vi "Dynamic Event Handler.vi"() -> ()   [LabVIEW 2013, in "Interaction By Refererence.lvclass"]
uses:
  Interaction By Refererence.lvclass
  Interaction By Refererence.lvclass/Interaction By Refererence.ctl
  IContainer/Interaction/Interaction.lvclass
panel:
  in  "Numeric 2":i32
  in  "Numeric":i32
  in  "Interaction":refnum<class "Interaction By Refererence.lvclass">
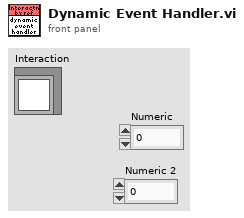
[diagram p1: front panel]
types:
  T1 = enum32{"Bad", "Idle", "Run top level", "Running"}
  T2 = typedef "LVRectTypeDef.ctl" = cluster{"Left":i16, "Top":i16, "Right":i16, "Bottom":i16}
  T3 = enum16{"VK_LBUTTON", "VK_RBUTTON", "VK_CANCEL", "VK_MBUTTON", "VK_XBUTTON1", "VK_XBUTTON2", "0x07", "VK_BACK", "VK_TAB", "0x0A", "0x0B", "VK_CLEAR", "VK_RETURN", "0x0E", "0x0F", "VK_SHIFT", "VK_CONTROL", "VK_MENU", "VK_PAUSE", "VK_CAPITAL", "VK_KANA\\VK_HANGUL", "0x16", "VK_JUNJA", "VK_FINAL", "VK_HANJA\\VK_KANJI", "0x1A", "VK_ESCAPE", "VK_CONVERT", "VK_NONCONVERT", "VK_ACCEPT", "VK_MODECHANGE", "VK_SPACE", "VK_PRIOR", "VK_NEXT", "VK_END", "VK_HOME", "VK_LEFT", "VK_UP", "VK_RIGHT", "VK_DOWN", "VK_SELECT", "VK_PRINT", "VK_EXECUTE", "VK_SNAPSHOT", "VK_INSERT", "VK_DELETE", "VK_HELP", "0 key", "1 key", "2 key", "3 key", "4 key", "5 key", "6 key", "7 key", "8 key", "9 key", "0x3A", "0x3B", "0x3C", "0x3D", "0x3E", "0x3F", "0x40", "A key", "B key", "C key", "D key", "E key", "F key", "G key", "H key", "I key", "J key", "K key", "L key", "M key", "N key", "O key", "P key", "Q key", "R key", "S key", "T key", "U key", "V key", "W key", "X key", "Y key", "Z key", "VK_LWIN", "VK_RWIN", "VK_APPS", "0x5E", "VK_SLEEP", "VK_NUMPAD0", "VK_NUMPAD1", "VK_NUMPAD2", "VK_NUMPAD3", "VK_NUMPAD4", "VK_NUMPAD5", "VK_NUMPAD6", "VK_NUMPAD7", "VK_NUMPAD8", "VK_NUMPAD9", "VK_MULTIPLY", "VK_ADD", "VK_SEPARATOR", "VK_SUBTRACT", "VK_DECIMAL", "VK_DIVIDE", "VK_F1", "VK_F2", "VK_F3", "VK_F4", "VK_F5", "VK_F6", "VK_F7", "VK_F8", "VK_F9", "VK_F10", "VK_F11", "VK_F12", "VK_F13", "VK_F14", "VK_F15", "VK_F16", "VK_F17", "VK_F18", "VK_F19", "VK_F20", "VK_F21", "VK_F22", "VK_F23", "VK_F24", "0x88", "0x89", "0x8A", "0x8B", "0x8C", "0x8D", "0x8E", "0x8F", "VK_NUMLOCK", "VK_SCROLL", "0x92", "0x93", "0x94", "0x95", "0x96", "0x97", "0x98", "0x99", "0x9A", "0x9B", "0x9C", "0x9D", "0x9E", "0x9F", "VK_LSHIFT", "VK_RSHIFT", "VK_LCONTROL", "VK_RCONTROL", "VK_LMENU", "VK_RMENU", "VK_BROWSER_BACK", "VK_BROWSER_FORWARD", "VK_BROWSER_REFRESH", "VK_BROWSER_STOP", "VK_BROWSER_SEARCH", "VK_BROWSER_FAVORITES", "VK_BROWSER_HOME", "VK_VOLUME_MUTE", "VK_VOLUME_DOWN", "VK_VOLUME_UP", "VK_MEDIA_NEXT_TRACK", "VK_MEDIA_PREV_TRACK", "VK_MEDIA_STOP", "VK_MEDIA_PLAY_PAUSE", "VK_LAUNCH_MAIL", "VK_LAUNCH_MEDIA_SELECT", "VK_LAUNCH_APP1", "VK_LAUNCH_APP2", "0xB8", "0xB9", "VK_OEM_1", "VK_OEM_PLUS", "VK_OEM_COMMA", "VK_OEM_MINUS", "VK_OEM_PERIOD", "VK_OEM_2", "VK_OEM_3", "0xC1", "0xC2", "0xC3", "0xC4", "0xC5", "0xC6", "0xC7", "0xC8", "0xC9", "0xCA", "0xCB", "0xCC", "0xCD", "0xCE", "0xCF", "0xD0", "0xD1", "0xD2", "0xD3", "0xD4", "0xD5", "0xD6", "0xD7", "0xD8", "0xD9", "0xDA", "VK_OEM_4", "VK_OEM_5", "VK_OEM_6", "VK_OEM_7", "VK_OEM_8", "0xE0", "0xE1", "VK_OEM_102", "0xE3", "0xE4", "VK_PROCESSKEY", "0xE6", "VK_PACKET", "0xE7", "0xE8", "0xE9", "0xEA", "0xEB", "0xEC", "0xED", "0xEF", "0xF0", "0xF1", "0xF2", "0xF3", "0xF4", "0xF5", "VK_ATTN", "VK_CRSEL", "VK_EXSEL", "VK_EREOF", "VK_PLAY", "VK_ZOOM", "VK_NONAME", "VK_PA1", "VK_OEM_CLEAR"}[]
  T4 = typedef "LVPoint32TypeDef.ctl" = cluster{"Horizontal":i32, "Vertical":i32}
  T5 = typedef "sizeaction.ctl" = enum32{"Minimized", "Maximized", "Resized"}
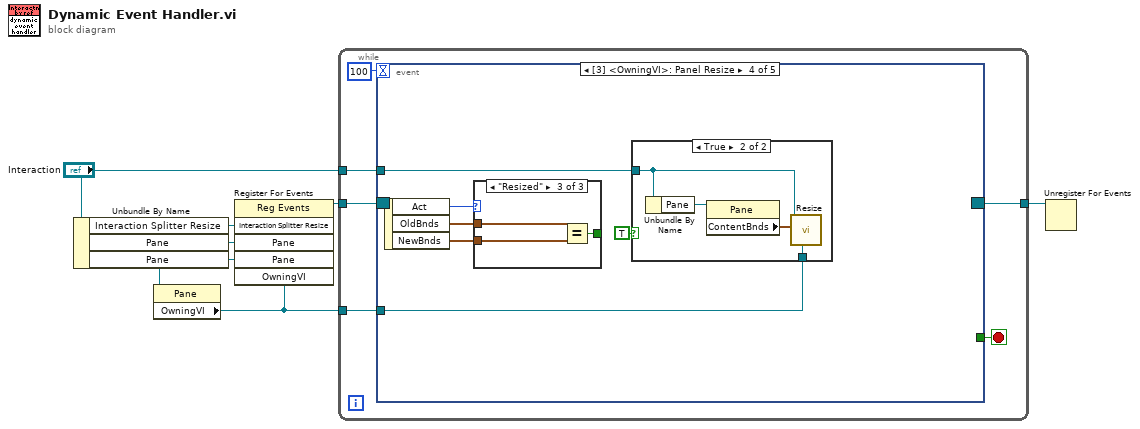
[diagram p0: block diagram]
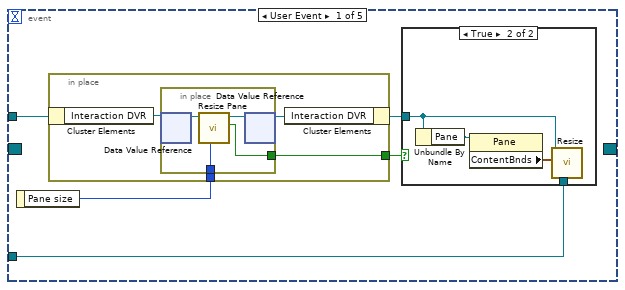
[diagram p2: hidden frame]
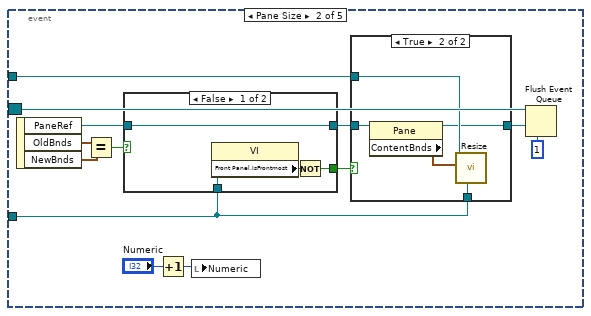
[diagram p4: hidden frame]
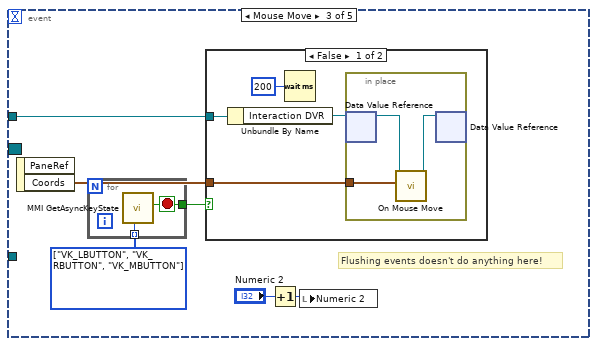
[diagram p7: hidden frame]
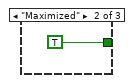
[diagram p11: hidden frame]
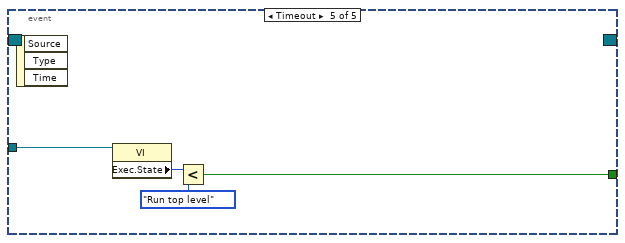
[diagram p12: hidden frame]
diagram:
  n1 = Unbundle By Name("Interaction") -> ("Interaction Splitter Resize"=w7:refnum<user-event>, "Pane"=w4:refnum<vi>, "Pane"=w3:refnum<vi>)
  n2 = property class="Pane"(reference=w3) -> ("OwningVI"=w2:refnum<vi>)  [unwired: 1 in, 2 out]
  n3 = register-events(w7, w4, w3, w2) -> (reference out=w6:refnum<event-registration>)  [unwired: 2 in, 1 out]
  n4 = while {
    tunnel: w6 -> [w12]
    tunnel: "Interaction" -> [w11]
    tunnel: w2 -> [w10]
    tunnel: [w8] -> w1
    stop <- w13 stop-if-true
    n5 = event shown="[3] <OwningVI>: Panel Resize" {
      selector: w12 -> [_ w36 _ _ _]
      dyn-events: [_ _ _ _ _] -> w8
      timeout: 100 -> [_ _ _ _ _]
      tunnel: [_ _ _ _ w85] -> w13
      tunnel: w11 -> [w16 w40 w59 w76 _]
      tunnel: w10 -> [w14 w31 _ w72 w88]
      event User Event {
        n6 = event-data() -> ("Pane size"=w15:i32)  [unwired: 1 in]
        n7 = in-place {
          in-place-border: [w22] -> w17
          in-place-border: w15 -> [w19]
          n8 = in-place-cluster #1(w16) -> ("Interaction DVR"=w20:refnum<data-value>)
          n9 = in-place {
            in-place-border: [w26] -> w22
            in-place-border: w19 -> [w23]
            n10 = in-place-dvr #2(w20) -> (w25:refnum<class "Interaction.lvclass">)  [unwired: 1 out]
            n11 = call-dynamic "Resize Pane.vi"("Pane size"=w23, "IContainer in"=w25) -> ("Resized?"=w26:bool, "IContainer out"=w24:refnum<class "Interaction.lvclass">)  [unwired: 7 in, 1 out]
            n12 = in-place-dvr #2(w24) -> (w21:refnum<data-value>)  [unwired: 1 out]
          }
          n13 = in-place-cluster #1("Interaction DVR"=w21) -> (w18:refnum<class "Interaction By Refererence.lvclass">)
        }
        n14 = case shown="True" w17 {
          tunnel: w18 -> [_ w29]
          tunnel: w14 -> [_ w27]
          frame False {
          }
          frame True {
            n15 = Unbundle By Name(w29) -> ("Pane"=w28:refnum<vi>)
            n16 = property on="Property Node" class="Pane"(reference=w28) -> ("ContentBnds"=w30:T2)  [unwired: 1 in, 2 out]
            n17 = call-dynamic "Resize.vi"("VI Refnum"=w27, "Bounds"=w30, "MMI Scaling in"=w29) -> ()  [unwired: 6 in, 3 out]
          }
        }
      }
      event Pane Size {
        n18 = event-data() -> ("PaneRef"=w37:refnum<vi>, "OldBnds"=w39:T2, "NewBnds"=w38:T2)  [unwired: 1 in]
        n19 = Equal?(x=w39, y=w38) -> (x = y?=w42:bool)
        n20 = case shown="False" w42 {
          selector: w42 -> [_ w49]
          tunnel: w37 -> [w44 w48]
          tunnel: [w44 w48] -> w41
          tunnel: [w47 w49] -> w43
          tunnel: w31 -> [w45 _]
          frame False {
            n21 = property on="Property Node" class="VI"(reference=w45) -> ("Front Panel.IsFrontmost"=w46:bool)  [unwired: 1 in, 2 out]
            n22 = Not(x=w46) -> (.not. x?=w47:bool)
          }
          frame True {
          }
        }
        n23 = Increment(x="Numeric") -> (x+1=w32:i32)
        n24 = local write "Numeric"(w32) -> ()
        n25 = case shown="True" w43 {
          tunnel: w40 -> [_ w53]
          tunnel: w41 -> [w50 w54]
          tunnel: [w50 w52] -> w34
          tunnel: w31 -> [_ w51]
          frame False {
          }
          frame True {
            n26 = property on="Property Node" class="Pane"(reference=w54) -> (reference out=w52:refnum<vi>, "ContentBnds"=w55:T2)  [unwired: 1 in, 1 out]
            n27 = call-dynamic "Resize.vi"("VI Refnum"=w51, "Bounds"=w55, "MMI Scaling in"=w53) -> ()  [unwired: 6 in, 3 out]
          }
        }
        n28 = Flush Event Queue(0:w36, 2:w34, 5:1 ("keep most recent")) -> ()  [unwired: 3 in, 3 out]
      }
      event Mouse Move {
        w61 = T3 [enum."VK_LBUTTON", enum."VK_RBUTTON", enum."VK_MBUTTON"] items=["VK_LBUTTON", "VK_RBUTTON", "VK_CANCEL", "VK_MBUTTON", "VK_XBUTTON1", "VK_XBUTTON2", "0x07", "VK_BACK", "VK_TAB", "0x0A", "0x0B", "VK_CLEAR", "VK_RETURN", "0x0E", "0x0F", "VK_SHIFT", "VK_CONTROL", "VK_MENU", "VK_PAUSE", "VK_CAPITAL", "VK_KANA\\VK_HANGUL", "0x16", "VK_JUNJA", "VK_FINAL", "VK_HANJA\\VK_KANJI", "0x1A", "VK_ESCAPE", "VK_CONVERT", "VK_NONCONVERT", "VK_ACCEPT", "VK_MODECHANGE", "VK_SPACE", "VK_PRIOR", "VK_NEXT", "VK_END", "VK_HOME", "VK_LEFT", "VK_UP", "VK_RIGHT", "VK_DOWN", "VK_SELECT", "VK_PRINT", "VK_EXECUTE", "VK_SNAPSHOT", "VK_INSERT", "VK_DELETE", "VK_HELP", "0 key", "1 key", "2 key", "3 key", "4 key", "5 key", "6 key", "7 key", "8 key", "9 key", "0x3A", "0x3B", "0x3C", "0x3D", "0x3E", "0x3F", "0x40", "A key", "B key", "C key", "D key", "E key", "F key", "G key", "H key", "I key", "J key", "K key", "L key", "M key", "N key", "O key", "P key", "Q key", "R key", "S key", "T key", "U key", "V key", "W key", "X key", "Y key", "Z key", "VK_LWIN", "VK_RWIN", "VK_APPS", "0x5E", "VK_SLEEP", "VK_NUMPAD0", "VK_NUMPAD1", "VK_NUMPAD2", "VK_NUMPAD3", "VK_NUMPAD4", "VK_NUMPAD5", "VK_NUMPAD6", "VK_NUMPAD7", "VK_NUMPAD8", "VK_NUMPAD9", "VK_MULTIPLY", "VK_ADD", "VK_SEPARATOR", "VK_SUBTRACT", "VK_DECIMAL", "VK_DIVIDE", "VK_F1", "VK_F2", "VK_F3", "VK_F4", "VK_F5", "VK_F6", "VK_F7", "VK_F8", "VK_F9", "VK_F10", "VK_F11", "VK_F12", "VK_F13", "VK_F14", "VK_F15", "VK_F16", "VK_F17", "VK_F18", "VK_F19", "VK_F20", "VK_F21", "VK_F22", "VK_F23", "VK_F24", "0x88", "0x89", "0x8A", "0x8B", "0x8C", "0x8D", "0x8E", "0x8F", "VK_NUMLOCK", "VK_SCROLL", "0x92", "0x93", "0x94", "0x95", "0x96", "0x97", "0x98", "0x99", "0x9A", "0x9B", "0x9C", "0x9D", "0x9E", "0x9F", "VK_LSHIFT", "VK_RSHIFT", "VK_LCONTROL", "VK_RCONTROL", "VK_LMENU", "VK_RMENU", "VK_BROWSER_BACK", "VK_BROWSER_FORWARD", "VK_BROWSER_REFRESH", "VK_BROWSER_STOP", "VK_BROWSER_SEARCH", "VK_BROWSER_FAVORITES", "VK_BROWSER_HOME", "VK_VOLUME_MUTE", "VK_VOLUME_DOWN", "VK_VOLUME_UP", "VK_MEDIA_NEXT_TRACK", "VK_MEDIA_PREV_TRACK", "VK_MEDIA_STOP", "VK_MEDIA_PLAY_PAUSE", "VK_LAUNCH_MAIL", "VK_LAUNCH_MEDIA_SELECT", "VK_LAUNCH_APP1", "VK_LAUNCH_APP2", "0xB8", "0xB9", "VK_OEM_1", "VK_OEM_PLUS", "VK_OEM_COMMA", "VK_OEM_MINUS", "VK_OEM_PERIOD", "VK_OEM_2", "VK_OEM_3", "0xC1", "0xC2", "0xC3", "0xC4", "0xC5", "0xC6", "0xC7", "0xC8", "0xC9", "0xCA", "0xCB", "0xCC", "0xCD", "0xCE", "0xCF", "0xD0", "0xD1", "0xD2", "0xD3", "0xD4", "0xD5", "0xD6", "0xD7", "0xD8", "0xD9", "0xDA", "VK_OEM_4", "VK_OEM_5", "VK_OEM_6", "VK_OEM_7", "VK_OEM_8", "0xE0", "0xE1", "VK_OEM_102", "0xE3", "0xE4", "VK_PROCESSKEY", "0xE6", "VK_PACKET", "0xE7", "0xE8", "0xE9", "0xEA", "0xEB", "0xEC", "0xED", "0xEF", "0xF0", "0xF1", "0xF2", "0xF3", "0xF4", "0xF5", "VK_ATTN", "VK_CRSEL", "VK_EXSEL", "VK_EREOF", "VK_PLAY", "VK_ZOOM", "VK_NONAME", "VK_PA1", "VK_OEM_CLEAR"]
        # "Flushing events doesn't do anything here!"
        n29 = event-data() -> ("Coords"=w58:T4)  [unwired: 1 in, 1 out]
        n30 = for {
          tunnel: [w63] -> w60
          tunnel: w61 -> [w62] mode=indexing
          stop <- w63 stop-if-true
          n31 = call "MMI GetAsyncKeyState.vi"("Enum"=w62) -> ("Pressed?"=w63:bool)  [unwired: 8 in, 2 out]
        }
        n32 = case shown="False" w60 {
          tunnel: w59 -> [w67 _]
          tunnel: w58 -> [w65 _]
          frame False {
            n33 = Unbundle By Name(w67) -> ("Interaction DVR"=w66:refnum<data-value>)
            n34 = Wait (ms)(milliseconds to wait=u32 200) -> ()  [unwired: 1 out]
            n35 = in-place {
              in-place-border: w65 -> [w70]
              n36 = in-place-dvr #3(w66) -> (w69:refnum<class "Interaction.lvclass">)  [unwired: 1 out]
              n37 = call "On Mouse Move.vi"("Coords"=w70, "Interaction in"=w69) -> ("Interaction out"=w68:refnum<class "Interaction.lvclass">)  [unwired: 8 in, 1 out]
              n38 = in-place-dvr #3(w68) -> ()  [unwired: 2 out]
            }
          }
          frame True {
          }
        }
        n39 = Increment(x="Numeric 2") -> (x+1=w56:i32)
        n40 = local write "Numeric 2"(w56) -> ()
      }
      event Panel Resize {
        n41 = event-data() -> ("Act"=w75:T5, "OldBnds"=w74:T2, "NewBnds"=w73:T2)  [unwired: 1 in]
        n42 = case shown="\"Resized\"" w75 {
          tunnel: [_ TRUE w84] -> _
          tunnel: w74 -> [_ _ w83]
          tunnel: w73 -> [_ _ w82]
          frame Default {
          }
          frame "Maximized" {
          }
          frame "Resized" {
            n43 = Equal?(x=w83, y=w82) -> (x = y?=w84:bool)
          }
        }
        n44 = case shown="True" TRUE {
          tunnel: w76 -> [_ w78]
          tunnel: w72 -> [_ w77]
          frame False {
          }
          frame True {
            n45 = Unbundle By Name(w78) -> ("Pane"=w79:refnum<vi>)
            n46 = property on="Property Node" class="Pane"(reference=w79) -> ("ContentBnds"=w80:T2)  [unwired: 1 in, 2 out]
            n47 = call-dynamic "Resize.vi"("VI Refnum"=w77, "Bounds"=w80, "MMI Scaling in"=w78) -> ()  [unwired: 6 in, 3 out]
          }
        }
      }
      event Timeout {
        n48 = event-data() -> ()  [unwired: 1 in, 3 out]
        n49 = property class="VI"(reference=w88) -> ("Exec.State"=w87:T1)  [unwired: 1 in, 2 out]
        n50 = Less?(x=w87, y=T1."Run top level" ("Execution:State")) -> (x < y?=w85:bool)
      }
    }
  }
  n51 = Unregister For Events(event registration refnum=w1) -> ()  [unwired: 1 in, 1 out]
